vi "FPGAcode2_test.vi"() -> ()   [LabVIEW 2015]
uses:
  <vilib>/Platform/TimedLoop/XDataNode/timing_clust.ctl
  <vilib>/Platform/TimedLoop/XDataNode/nitl_modes.ctl
  <vilib>/Platform/TimedLoop/XDataNode/wakeup.ctl
  <vilib>/rvi/Emulation/niFpgaGetClockAttributes.vi
  <vilib>/rvi/Emulation/niFpgaSctlEmulationGetInTimedLoop.vi
  <vilib>/rvi/Emulation/niFpgaEmulationReportErrorSimple.vi
  <vilib>/rvi/Emulation/niFpgaProcessEmulError.vi
  <vilib>/rvi/eio/common/nirviEmuTemplateMethod_errors.vi
  <vilib>/rvi/Emulation/niFpgaCriticalErrorInLSC.vi
  <vilib>/eio/EIONode/EIONode.xnode
  <vilib>/Platform/TimedLoop/XDataNode/XDataNode.xnode
  <vilib>/Platform/TimedLoop/XDataNode/XDNodeRunTimeDep.lvlib
panel:
  out "New Average":T1
  in  "Cluster":T1
  out "Detector 3 Correlation 7":i16
  out "Detector 3 Correlation 6":i16
  out "Detector 3 Correlation 5":i16
  out "Detector 3 Correlation 4":i16
  out "Detector 3 Correlation 3":i16
  out "Detector 3 Correlation 2":i16
  out "Detector 3 Correlation 1":i16
  out "Detector 1 Correlation 7":i16
  out "Detector 1 Correlation 6":i16
  out "Detector 1 Correlation 5":i16
  out "Detector 1 Correlation 4":i16
  out "Detector 1 Correlation 3":i16
  out "Detector 1 Correlation 2":i16
  out "Detector 1 Correlation 1":i16
  in  "Filter threshold 7":i32=1000
  in  "Filter threshold 6":i32=1000
  in  "Filter threshold 5":i32=1000
  in  "Filter threshold 4":i32=1000
  in  "Filter threshold 3":i32=1000
  in  "Filter threshold 2":i32=1000
  in  "Filter threshold 1":i32=1000
  out "Del Armed":bool
  out "Armed":bool
  out "Delay":bool
  out "Plates":bool
  in  "Reset One Shot":bool
  in  "One Shot":bool
  in  "High Charge Limit":i16
  in  "Low Charge Limit":i16
  in  "High Velocity Count":i32
  in  "Low Velocity Count":i32
  in  "High Mass Limit":i64
  in  "Low Mass Limit":i64
  in  "Mult1":fxp<+,16,7>
  out "IO Module\\AI 0":i16
  out "IO Module\\AI 1":i16
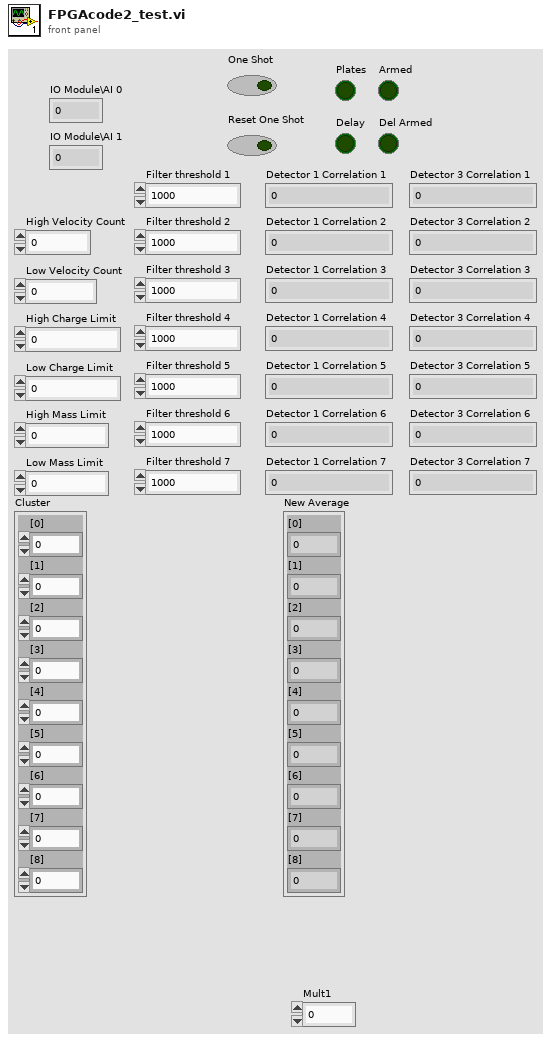
[diagram p1: front panel]
types:
  T1 = cluster{"[0]":i32, "[1]":i32, "[2]":i32, "[3]":i32, "[4]":i32, "[5]":i32, "[6]":i32, "[7]":i32, "[8]":i32}
  T2 = typedef "XDNodeRunTimeDep.lvlib/timing_clust.ctl" = cluster{"Expected End [f-1]":u64, "Actual End [f-1]":u64, "Finished Late? [f-1]":bool, "Expected End [i-1]":u64, "Actual End [i-1]":u64, "Finished Late? [i-1]":bool, "Expected Start [i]":u64, "Actual Start [i]":u64, "Expected Start [f]":u64, "Actual Start [f]":u64, "Source Name":string, "Structure Name":string, "Period":i64, "Deadline":i64, "Offset":i64, "Start":i64, "Priority":i32, "Timeout":i32, "Mode":T3, "Wakeup Reason":T4, "Error":errorcluster, "Source Type":string, "Secondary Source Type":string, "Global End Time":u64, "Global Start Time":u64, "Frame Duration":u64, "Iteration Duration":u64, "Assigned CPU":i32, "I/O Scan Engine Mode":u32}
  T3 = typedef "XDNodeRunTimeDep.lvlib/nitl_modes.ctl" = enum32{"No Change", "Process missed periods, maintain original phase", "Discard missed periods, maintain original phase", "Process missed periods, ignore original phase", "Discard missed periods, ignore original phase"}
  T4 = typedef "XDNodeRunTimeDep.lvlib/wakeup.ctl" = enum32{"Normal", "Aborted", "Asynchronous wakeup", "Timing source error", "Timed loop error", "Timeout"}
  T5 = cluster{"[0]":u8, "[1]":u8, "[2]":u8, "[3]":u8, "[4]":u8, "[5]":u8, "[6]":u8, "[7]":u8, "[8]":u8}
  T6 = cluster{"High Charge Limit":i16, "Low Charge Limit":i16, "Time Out Limit":i32, "High Velocity Count":i32, "Low Velocity Count":i32, "Sampling Rate":fxp<+,30,25>, "High Mass Limit":i64, "Low Mass Limit":i64}
  T7 = cluster{"[0]":u32, "[1]":u32, "[2]":u32, "[3]":u32, "[4]":u32, "[5]":u32, "[6]":u32, "[7]":u32, "[8]":u32}
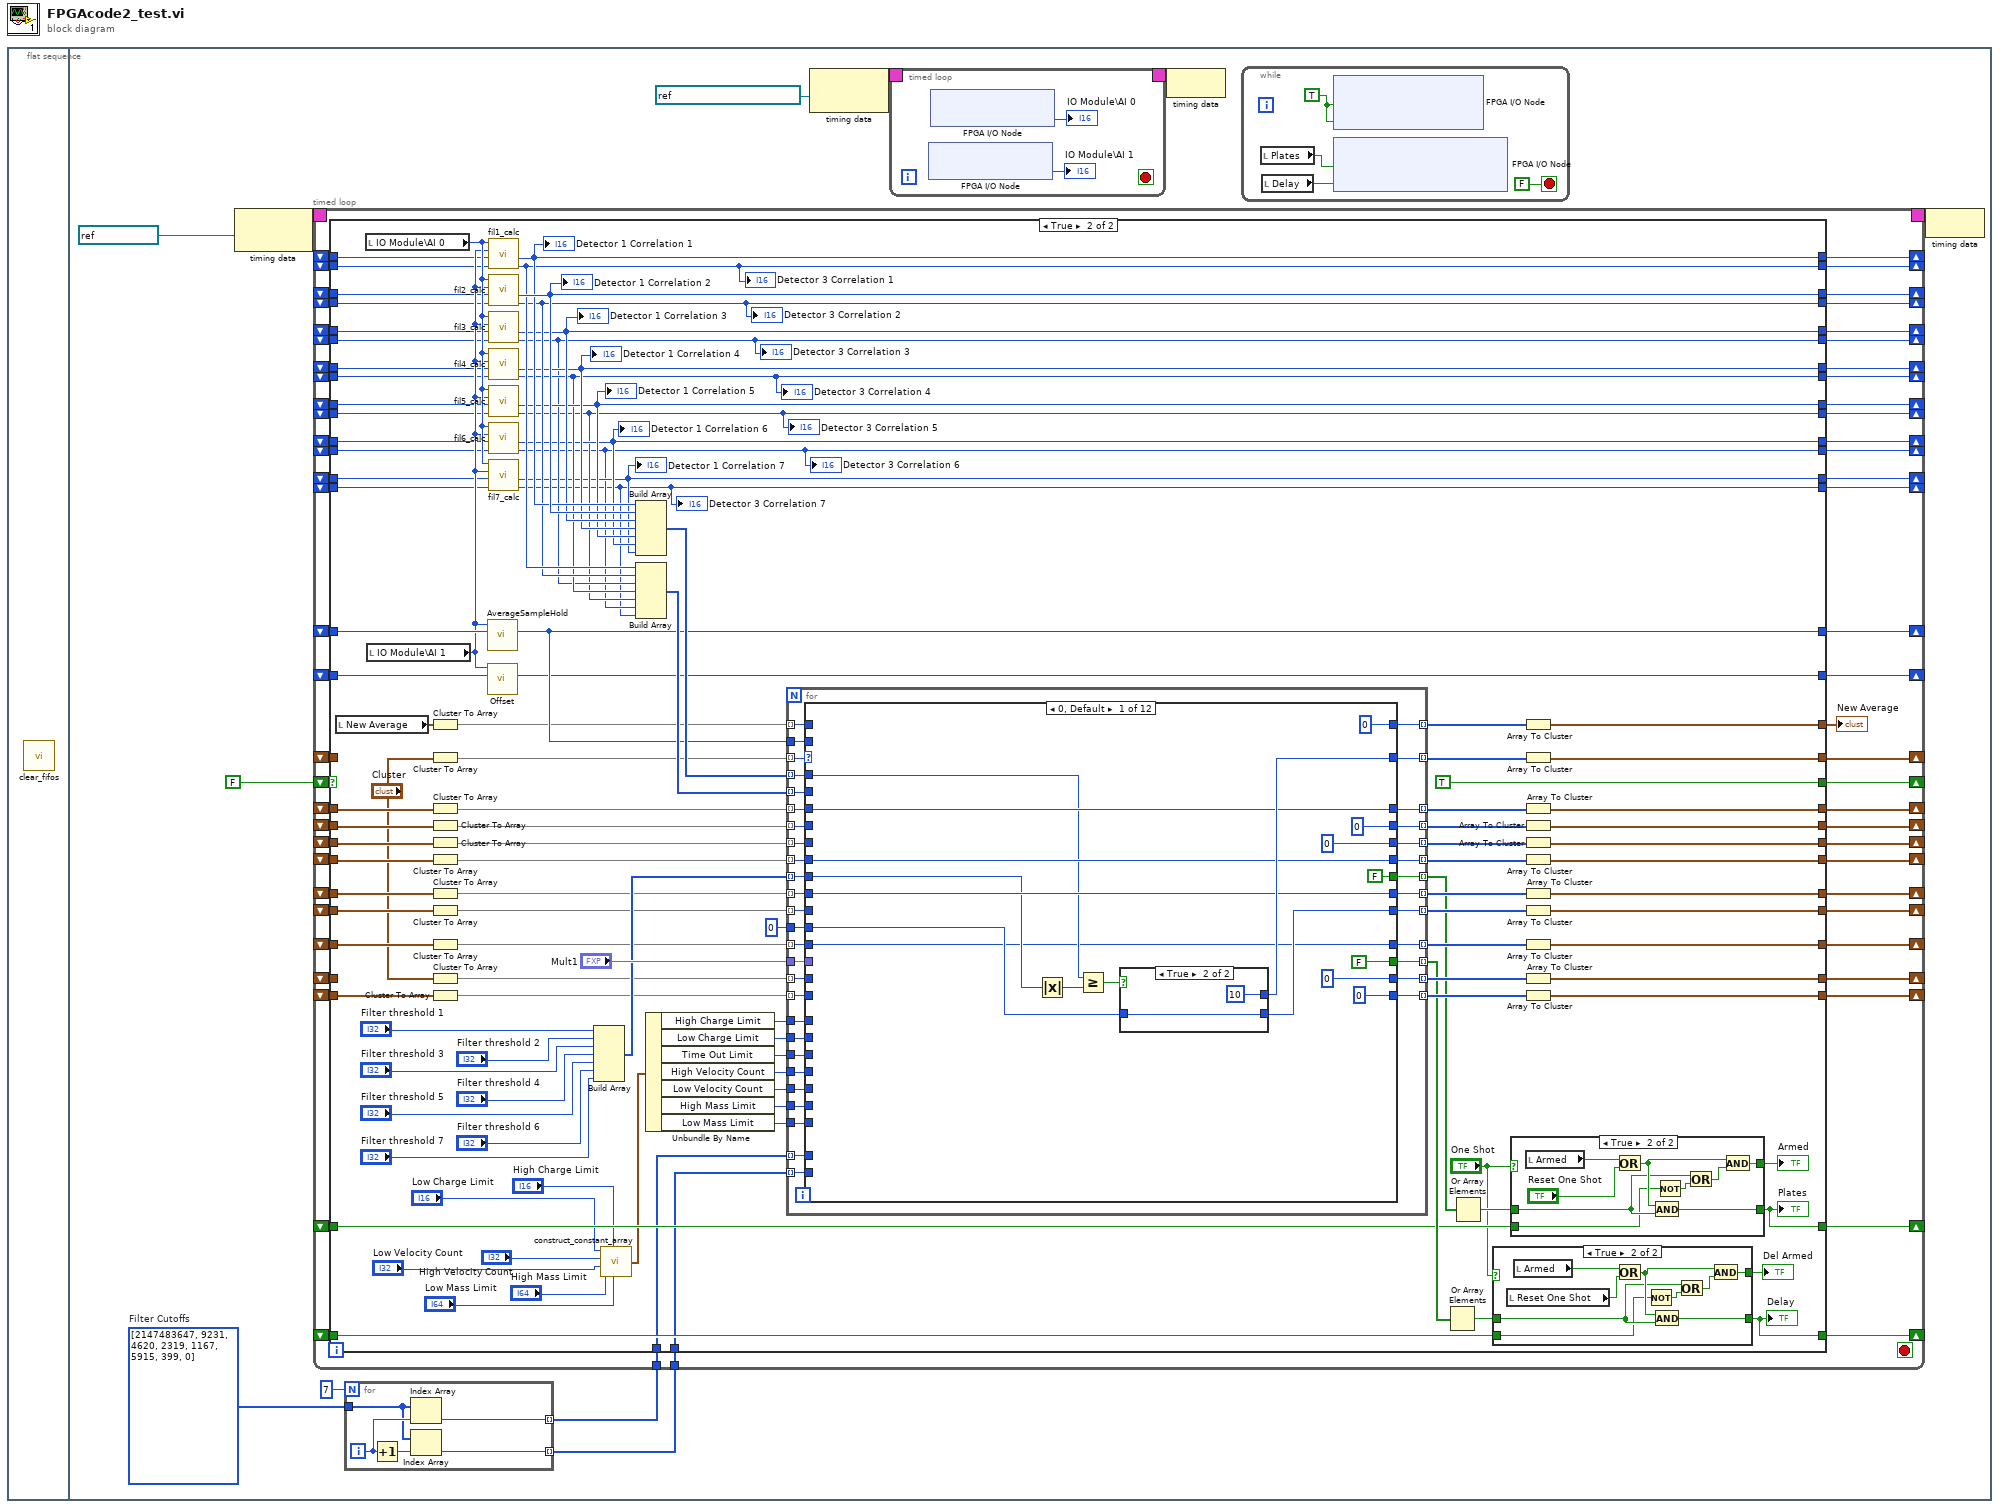
[diagram p0: block diagram]
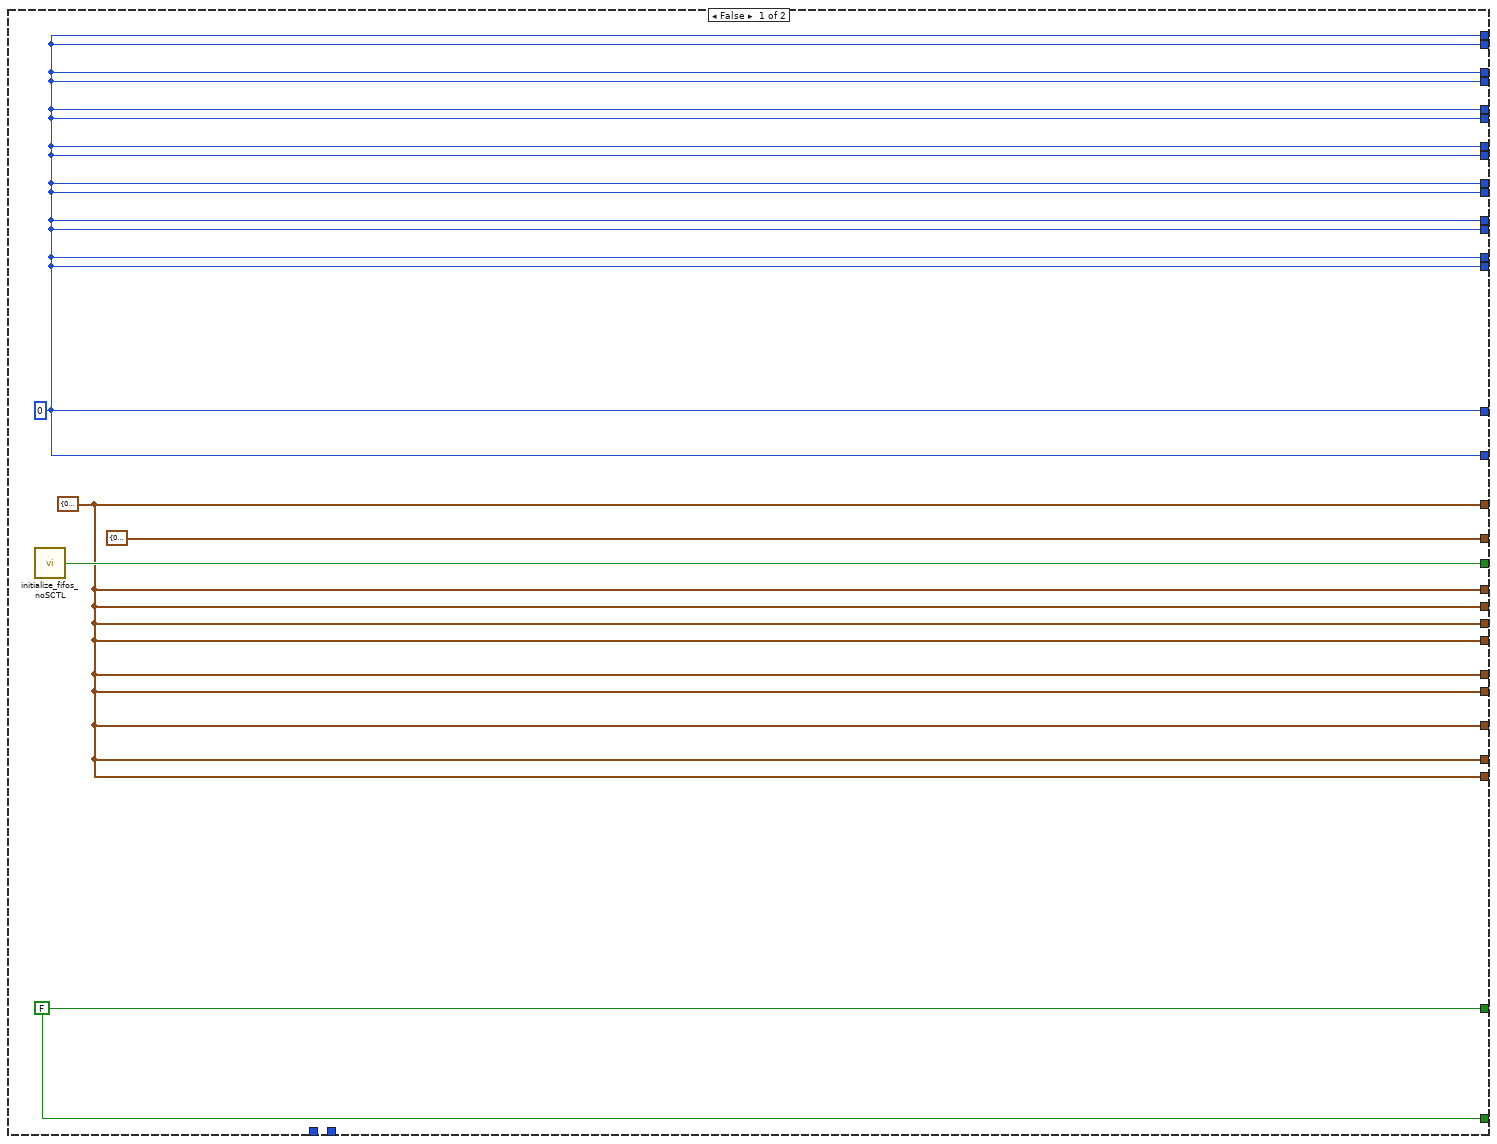
[diagram p2: hidden frame]
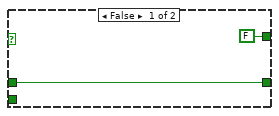
[diagram p3: hidden frame]
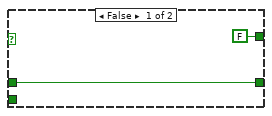
[diagram p4: hidden frame]
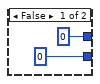
[diagram p5: hidden frame]
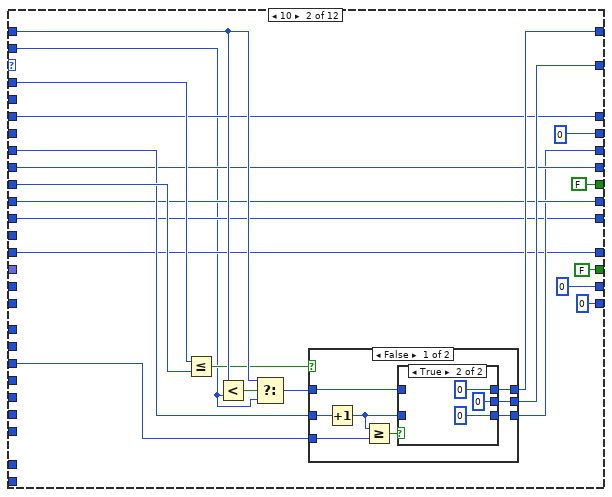
[diagram p6: hidden frame]
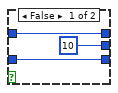
[diagram p7: hidden frame]
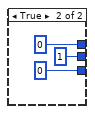
[diagram p8: hidden frame]
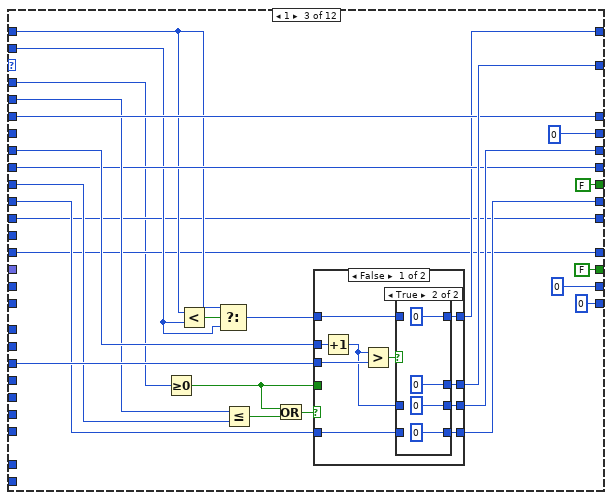
[diagram p9: hidden frame]
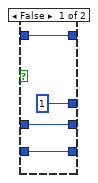
[diagram p10: hidden frame]
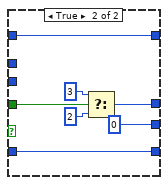
[diagram p11: hidden frame]
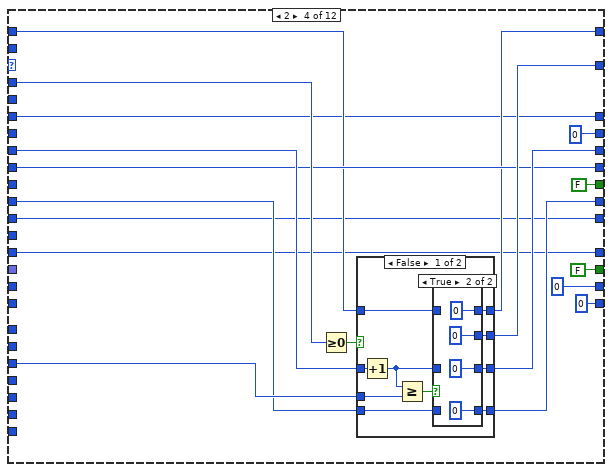
[diagram p12: hidden frame]
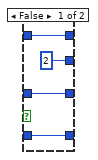
[diagram p13: hidden frame]
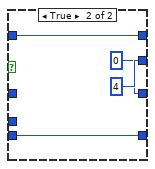
[diagram p14: hidden frame]
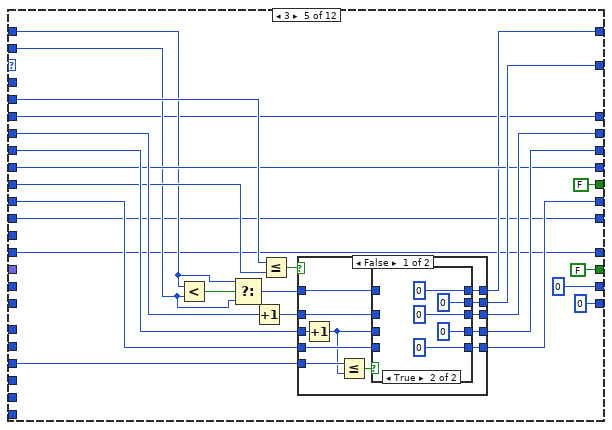
[diagram p15: hidden frame]
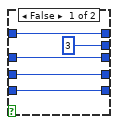
[diagram p16: hidden frame]
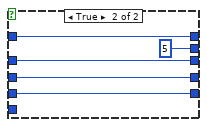
[diagram p17: hidden frame]
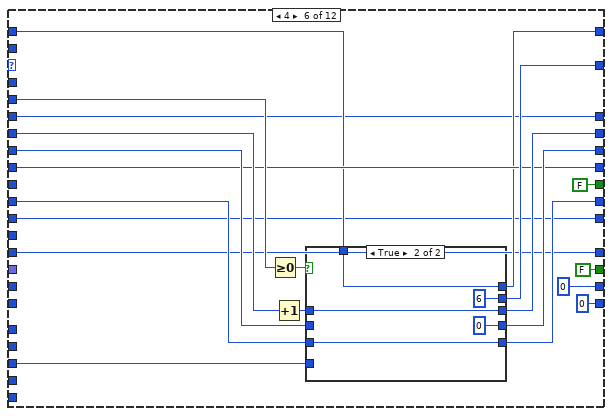
[diagram p18: hidden frame]
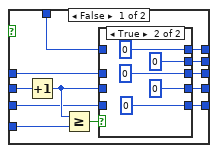
[diagram p19: hidden frame]
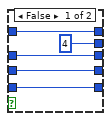
[diagram p20: hidden frame]
diagram:
  n1 = flat-sequence {
    frame #0 {
      n2 = call "clear_fifos.vi"() -> ()  [unwired: 1 in]
    }
    frame #1 {
      w3 = i32[] [2147483647, 9231, 4620, 2319, 1167, 5915, 399, 0]  # Filter Cutoffs
      n3 = node-c288(refnum<k21> "26.67MHz" ("Source Name")) -> (w11:T2)
      n4 = for {
        N: 7 -> [_]
        tunnel: w3 -> [w14]
        tunnel: [w13] -> w2 mode=indexing
        tunnel: [w12] -> w1 mode=indexing
        i -> [w16]
        n5 = Increment(x=w16) -> (x+1=w15:i32)
        n6 = Index Array(array=w14, index=w16) -> (element=w13:i32)
        n7 = Index Array(array=w14, index=w15) -> (element=w12:i32)
      }
      n8 = timed-loop {
        timing: w11 -> [_]
        timing-out: [_] -> w10
        shift-right: [w88] -> _
        shift-left: FALSE -> [w89]
        shift-right: [w86] -> _
        shift-left: _ -> [w87]
        shift-right: [w84] -> _
        shift-left: _ -> [w85]
        shift-right: [w70] -> _
        shift-left: _ -> [w83]
        shift-right: [w81] -> _
        shift-left: _ -> [w82]
        shift-right: [w79] -> _
        shift-left: _ -> [w80]
        shift-right: [w69] -> _
        shift-left: _ -> [w78]
        shift-right: [w68] -> _
        shift-left: _ -> [w77]
        shift-right: [w64] -> _
        shift-left: _ -> [w76]
        shift-right: [w74] -> _
        shift-left: _ -> [w75]
        shift-right: [w67] -> _
        shift-left: _ -> [w73]
        shift-right: [w66] -> _
        shift-left: _ -> [w72]
        shift-right: [w65] -> _
        shift-left: _ -> [w71]
        shift-right: [w63] -> _
        shift-left: _ -> [w62]
        shift-right: [w60] -> _
        shift-left: _ -> [w61]
        shift-right: [w59] -> _
        shift-left: _ -> [w58]
        shift-right: [w57] -> _
        shift-left: _ -> [w56]
        shift-right: [w55] -> _
        shift-left: _ -> [w51]
        shift-right: [w54] -> _
        shift-left: _ -> [w50]
        shift-right: [w53] -> _
        shift-left: _ -> [w49]
        shift-right: [w52] -> _
        shift-left: _ -> [w48]
        shift-right: [w47] -> _
        shift-left: _ -> [w39]
        shift-right: [w46] -> _
        shift-left: _ -> [w38]
        shift-right: [w45] -> _
        shift-left: _ -> [w37]
        shift-right: [w44] -> _
        shift-left: _ -> [w32]
        shift-right: [w43] -> _
        shift-left: _ -> [w36]
        shift-right: [w42] -> _
        shift-left: _ -> [w33]
        shift-right: [w41] -> _
        shift-left: _ -> [w35]
        shift-right: [w40] -> _
        shift-left: _ -> [w34]
        tunnel: w2 -> [w31]
        tunnel: w1 -> [w30]
        stop <- _ stop-if-true
        n9 = case shown="True" w89 {
          tunnel: [w94 TRUE] -> w88
          tunnel: [w90 w121] -> w29
          tunnel: w87 -> [_ w209]
          tunnel: [w92 w146] -> w86
          tunnel: w85 -> [_ _]
          tunnel: [T5 {"[0]"=0, "[1]"=0, "[2]"=0, "[3]"=0, "[4]"=0, "[5]"=0, "[6]"=0, "[7]"=0, "[8]"=0} w120] -> w84
          tunnel: w83 -> [_ w207]
          tunnel: w82 -> [_ w97]
          tunnel: [w90 w111] -> w81
          tunnel: w80 -> [_ _]
          tunnel: [w90 w112] -> w79
          tunnel: w78 -> [_ w204]
          tunnel: w77 -> [_ w203]
          tunnel: w76 -> [_ w202]
          tunnel: w75 -> [_ w201]
          tunnel: [w92 w99] -> w74
          tunnel: w73 -> [_ w200]
          tunnel: w72 -> [_ w199]
          tunnel: w71 -> [_ w198]
          tunnel: [w90 w119] -> w70
          tunnel: [w90 w118] -> w69
          tunnel: [w90 w117] -> w68
          tunnel: [w90 w116] -> w67
          tunnel: [w90 w115] -> w66
          tunnel: [w90 w114] -> w65
          tunnel: [w90 w113] -> w64
          tunnel: [w93 w185] -> w63
          tunnel: w62 -> [_ w186]
          tunnel: w61 -> [_ w182]
          tunnel: [w93 w181] -> w60
          tunnel: [w92 w132] -> w59
          tunnel: w58 -> [_ w160]
          tunnel: [w92 w134] -> w57
          tunnel: w56 -> [_ w159]
          tunnel: [w92 w133] -> w55
          tunnel: [w92 w136] -> w54
          tunnel: [w92 w135] -> w53
          tunnel: [w92 w139] -> w52
          tunnel: w51 -> [_ w158]
          tunnel: w50 -> [_ w157]
          tunnel: w49 -> [_ w156]
          tunnel: w48 -> [_ w155]
          tunnel: [w92 w138] -> w47
          tunnel: [w92 w140] -> w46
          tunnel: [w92 w137] -> w45
          tunnel: [w92 w141] -> w44
          tunnel: [w92 w142] -> w43
          tunnel: [w92 w145] -> w42
          tunnel: [w92 w143] -> w41
          tunnel: [w92 w144] -> w40
          tunnel: w39 -> [_ w154]
          tunnel: w38 -> [_ w153]
          tunnel: w37 -> [_ w152]
          tunnel: w36 -> [_ w151]
          tunnel: w35 -> [_ w150]
          tunnel: w34 -> [_ w149]
          tunnel: w33 -> [_ w148]
          tunnel: w32 -> [_ w147]
          tunnel: w31 -> [_ w131]
          tunnel: w30 -> [_ w130]
          frame False {
            w90 = T1 {"[0]"=0, "[1]"=0, "[2]"=0, "[3]"=0, "[4]"=0, "[5]"=0, "[6]"=0, "[7]"=0, "[8]"=0}
            w93 = FALSE
            w92 = i16 0 ("Output New Average")
            n10 = call "initialize_fifos_noSCTL.vi"() -> ("Output State"=w94:bool)
          }
          frame True {
            n11 = local read "New Average"() -> (w95:T1)
            n12 = local read "IO Module\\AI 0"() -> (w172:i16)
            n13 = local read "IO Module\\AI 1"() -> (w171:i16)
            n14 = Cluster To Array(cluster=w95) -> (array=w110:i32[])
            n15 = Cluster To Array(cluster="Cluster") -> (array=w109:i32[])
            n16 = Cluster To Array(cluster=w207) -> (array=w108:i32[])
            n17 = Cluster To Array(cluster=w204) -> (array=w107:i32[])
            n18 = Cluster To Array(cluster=w203) -> (array=w106:u32[])
            n19 = Cluster To Array(cluster=w200) -> (array=w105:i32[])
            n20 = Cluster To Array(cluster=w199) -> (array=w104:i32[])
            n21 = Cluster To Array(cluster=w198) -> (array=w103:i32[])
            n22 = Cluster To Array(cluster=w202) -> (array=w102:i32[])
            n23 = Cluster To Array(cluster="Cluster") -> (array=w101:i32[])
            n24 = Cluster To Array(cluster=w97) -> (array=w100:i32[])
            n25 = call "AverageSampleHold.vi"("Previous Average"=w209, "Input Value"=w171) -> ("Output New Average"=w146:i16)  [unwired: 9 in]
            n26 = call "Offset.vi"("Previous Average"=w201, "Input Value"=w171) -> ("Output New Average"=w99:i16)  [unwired: 9 in]
            n27 = call "fil1_calc.vi"("Detector 3 Correlation In"=w150, "Detector 1 Correlation In"=w149, "AI1"=w171, "AI0"=w172) -> ("Detector 3 Correlation Out"=w143:i16, "Detector 1 Correlation Out"=w144:i16)  [unwired: 4 in]
            "Detector 1 Correlation 1" <- w144
            "Detector 3 Correlation 1" <- w143
            n28 = call "fil2_calc.vi"("Detector 3 Correlation In"=w151, "Detector 1 Correlation In"=w148, "AI1"=w171, "AI0"=w172) -> ("Detector 3 Correlation Out"=w142:i16, "Detector 1 Correlation Out"=w145:i16)  [unwired: 4 in]
            "Detector 1 Correlation 2" <- w145
            "Detector 3 Correlation 2" <- w142
            n29 = call "fil3_calc.vi"("Detector 3 Correlation In"=w152, "Detector 1 Correlation In"=w147, "AI1"=w171, "AI0"=w172) -> ("Detector 3 Correlation Out"=w137:i16, "Detector 1 Correlation Out"=w141:i16)  [unwired: 4 in]
            "Detector 1 Correlation 3" <- w141
            "Detector 3 Correlation 3" <- w137
            n30 = call "fil4_calc.vi"("Detector 3 Correlation In"=w154, "Detector 1 Correlation In"=w153, "AI1"=w171, "AI0"=w172) -> ("Detector 3 Correlation Out"=w138:i16, "Detector 1 Correlation Out"=w140:i16)  [unwired: 4 in]
            "Detector 1 Correlation 4" <- w140
            "Detector 3 Correlation 4" <- w138
            n31 = call "fil5_calc.vi"("Detector 3 Correlation In"=w156, "Detector 1 Correlation In"=w155, "AI1"=w171, "AI0"=w172) -> ("Detector 3 Correlation Out"=w135:i16, "Detector 1 Correlation Out"=w139:i16)  [unwired: 4 in]
            "Detector 1 Correlation 5" <- w139
            "Detector 3 Correlation 5" <- w135
            n32 = call "fil6_calc.vi"("Detector 3 Correlation In"=w158, "Detector 1 Correlation In"=w157, "AI1"=w171, "AI0"=w172) -> ("Detector 3 Correlation Out"=w133:i16, "Detector 1 Correlation Out"=w136:i16)  [unwired: 4 in]
            "Detector 1 Correlation 6" <- w136
            "Detector 3 Correlation 6" <- w133
            n33 = call "fil7_calc.vi"("Detector 3 Correlation In"=w160, "Detector 1 Correlation In"=w159, "AI1"=w171, "AI0"=w172) -> ("Detector 3 Correlation Out"=w132:i16, "Detector 1 Correlation Out"=w134:i16)  [unwired: 4 in]
            "Detector 1 Correlation 7" <- w134
            "Detector 3 Correlation 7" <- w132
            n34 = Build Array("Filter threshold 1", "Filter threshold 2", "Filter threshold 3", "Filter threshold 4", "Filter threshold 5", "Filter threshold 6", "Filter threshold 7") -> (w161:i32[])
            n35 = call "construct_constant_array.vi"("Low Mass Limit"="Low Mass Limit", "High Charge Limit"="High Charge Limit", "High Mass Limit"="High Mass Limit", "Low Velocity Count"="Low Velocity Count", "High Velocity Count"="High Velocity Count", "Low Charge Limit"="Low Charge Limit") -> ("Limits"=w129:T6)
            n36 = Build Array(w144, w145, w141, w140, w139, w136, w134) -> (w170:i16[])
            n37 = Build Array(w143, w142, w137, w138, w135, w133, w132) -> (w169:i16[])
            n38 = Unbundle By Name(w129) -> ("High Charge Limit"=w122:i16, "Low Charge Limit"=w123:i16, "Time Out Limit"=w124:i32, "High Velocity Count"=w125:i32, "Low Velocity Count"=w126:i32, "High Mass Limit"=w127:i64, "Low Mass Limit"=w128:i64)
            n39 = for {
              tunnel: w170 -> [w269] mode=indexing
              tunnel: w169 -> [w268] mode=indexing
              tunnel: w110 -> [w272] mode=indexing
              tunnel: [w253] -> w210 mode=indexing
              tunnel: w109 -> [w270] mode=indexing
              tunnel: [w252] -> w208 mode=indexing
              tunnel: w108 -> [w267] mode=indexing
              tunnel: w100 -> [w256] mode=indexing
              tunnel: [w241] -> w206 mode=indexing
              tunnel: w101 -> [w257] mode=indexing
              tunnel: [w242] -> w205 mode=indexing
              tunnel: w107 -> [w266] mode=indexing
              tunnel: w106 -> [w265] mode=indexing
              tunnel: w102 -> [w259] mode=indexing
              tunnel: w105 -> [w264] mode=indexing
              tunnel: w161 -> [w263] mode=indexing
              tunnel: w104 -> [w262] mode=indexing
              tunnel: w103 -> [w261] mode=indexing
              tunnel: [w251] -> w197 mode=indexing
              tunnel: [w250] -> w196 mode=indexing
              tunnel: [w249] -> w195 mode=indexing
              tunnel: [w248] -> w194 mode=indexing
              tunnel: [w245] -> w193 mode=indexing
              tunnel: [w244] -> w192 mode=indexing
              tunnel: [w243] -> w191 mode=indexing
              tunnel: [w247] -> w190 mode=indexing
              tunnel: [w246] -> w189 mode=indexing
              tunnel: "Mult1" -> [w258]
              tunnel: w146 -> [w271]
              tunnel: i16 0 ("Output New Average") -> [w260]
              tunnel: w131 -> [w255] mode=indexing
              tunnel: w130 -> [w254] mode=indexing
              tunnel: w128 -> [w240]
              tunnel: w127 -> [w239]
              tunnel: w126 -> [w238]
              tunnel: w125 -> [w237]
              tunnel: w124 -> [w236]
              tunnel: w123 -> [w235]
              tunnel: w122 -> [w234]
              n40 = case shown="0, Default" w270 {
                tunnel: w269 -> [w283 w314 w334 w399 _ _ _ _ _ _ _ _]
                tunnel: w268 -> [_ _ w351 _ w442 w490 w537 _ _ _ _ _]
                tunnel: w263 -> [w281 w313 w350 _ w441 _ _ _ _ _ _ _]
                tunnel: w266 -> [_ _ _ _ w444 w498 w546 w589 w646 w675 w705 _]
                tunnel: [0 0 0 0 w450 w496 w539 w574 w645 w673 w703 0] -> w250
                tunnel: [w290 w311 w359 w403 w449 w493 w542 w594 w644 w674 w704 w729] -> w252
                tunnel: w267 -> [w287 w306 w352 w390 w430 w482 w538 w595 w620 w659 w701 w720]
                tunnel: w236 -> [_ w309 w358 w402 w447 w491 w543 _ _ _ _ _]
                tunnel: w265 -> [_ w310 w357 w401 w448 w492 w545 _ _ _ _ _]
                tunnel: [u32 0 w301 w356 w400 w446 w494 w541 u32 0 u32 0 ("Timeout Count in") u32 0 ("Timeout Count in") u32 0 u32 0 ("Timeout Count in")] -> w249
                tunnel: w238 -> [_ _ _ _ _ _ _ _ w643 _ _ _]
                tunnel: w237 -> [_ _ _ _ _ _ _ _ w642 _ _ _]
                tunnel: [w287 w306 w352 w390 w430 w482 w538 w596 w620 w659 w701 w720] -> w251
                tunnel: w235 -> [_ _ _ _ _ _ _ _ w641 _ _ _]
                tunnel: w234 -> [_ _ _ _ _ _ _ _ w640 _ _ _]
                tunnel: w262 -> [w286 w303 w349 w397 w440 w485 w536 w592 w639 w671 w699 _]
                tunnel: [w286 w303 w348 w396 w439 w489 w535 w593 w638 w671 w700 0 ("Noise Level")] -> w245
                tunnel: w264 -> [w285 w304 w347 w395 w438 w488 w534 w591 w621 w667 w696 w722]
                tunnel: [w285 w304 w347 w395 w438 w488 w534 w591 w621 w668 w696 w722] -> w248
                tunnel: [0 ("Old Average In") w307 w346 w394 w437 w487 w533 w590 w634 w664 0 ("Old Average In") 0 ("Old Average In")] -> w253
                tunnel: w255 -> [_ _ _ _ _ _ _ w576 _ _ _ _]
                tunnel: w254 -> [_ _ _ _ _ _ _ w575 _ _ _ _]
                tunnel: [FALSE FALSE ("Data") FALSE FALSE FALSE FALSE FALSE FALSE FALSE ("Data") w658 w690 FALSE ("Data")] -> w247
                tunnel: w272 -> [_ w315 w343 w392 w434 w484 w531 w586 w634 w664 _ _]
                tunnel: w271 -> [_ w295 w342 _ w433 _ _ _ _ _ _ _]
                tunnel: w261 -> [_ w300 w340 w391 w431 w483 w530 w585 w635 w663 _ _]
                tunnel: w260 -> [w278 _ _ _ _ _ _ _ _ _ _ _]
                tunnel: [w279 w300 w340 w391 w431 w483 w530 w585 w635 w663 0 ("Offset") 0 ("Offset")] -> w244
                tunnel: [w277 w299 w339 w389 w429 w481 w529 w584 w622 w669 w694 w727] -> w243
                tunnel: w259 -> [w277 w299 w339 w389 w429 w481 w529 w584 w622 w670 w694 w727]
                tunnel: w239 -> [_ _ _ _ _ _ _ _ w633 _ _ _]
                tunnel: w240 -> [_ _ _ _ _ _ _ _ w632 _ _ _]
                tunnel: w257 -> [_ _ _ _ _ _ _ _ w628 w662 w693 w718]
                tunnel: [0 0 0 0 0 0 0 w580 w627 w660 w688 w715] -> w241
                tunnel: [FALSE FALSE FALSE FALSE FALSE FALSE FALSE FALSE FALSE w657 w689 w719] -> w246
                tunnel: [u16 0 u16 0 u16 0 u16 0 u16 0 u16 0 u16 0 u16 0 u16 0 u16 0 w692 w728] -> w242
                tunnel: w256 -> [_ _ _ _ _ _ _ _ _ _ _ w716]
                tunnel: w258 -> [_ _ _ _ _ _ _ w579 _ _ _ _]
                frame 0, Default {
                  n41 = Absolute Value(x=w281) -> (abs(x)=w280:i32)
                  n42 = Greater Or Equal?(x=w283, y=w280) -> (x >= y?=w288:bool)
                  n43 = case shown="True" w288 {
                    tunnel: [u8 0 u8 10] -> w290
                    tunnel: [0 w293] -> w279
                    tunnel: w278 -> [_ w293]
                    frame False {
                    }
                    frame True {
                    }
                  }
                }
                frame 10 {
                  n44 = Less Or Equal?(x=w314, y=w313) -> (x <= y?=w312:bool)
                  n45 = Less?(x=w315, y=w295) -> (x < y?=w316:bool)
                  n46 = Select(t=w315, s=w316, f=w295) -> (s? t:f=w308:i32)
                  n47 = case shown="False" w312 {
                    tunnel: [w322 u8 1] -> w311
                    tunnel: w310 -> [w319 _]
                    tunnel: w309 -> [w324 _]
                    tunnel: w308 -> [w321 _]
                    tunnel: [w320 0 ("New Average")] -> w307
                    tunnel: [w317 0] -> w301
                    frame False {
                      n48 = Increment(x=w319) -> (x+1=w318:u32)
                      n49 = Greater Or Equal?(x=w318, y=w324) -> (x >= y?=w323:bool)
                      n50 = case shown="True" w323 {
                        tunnel: [u8 10 u8 0] -> w322
                        tunnel: w321 -> [w327 _]
                        tunnel: [w327 0 ("New Average")] -> w320
                        tunnel: w318 -> [w325 _]
                        tunnel: [w325 0] -> w317
                        frame False {
                        }
                        frame True {
                        }
                      }
                    }
                    frame True {
                    }
                  }
                }
                frame 1 {
                  n51 = Greater Or Equal To 0?(x=w334) -> (x >= 0?=w354:bool)
                  n52 = Less?(x=w343, y=w342) -> (x < y?=w344:bool)
                  n53 = Select(t=w343, s=w344, f=w342) -> (s? t:f=w341:i32)
                  n54 = Less Or Equal?(x=w351, y=w350) -> (x <= y?=w353:bool)
                  n55 = Or(x=w354, y=w353) -> (x .or. y?=w355:bool)
                  n56 = case shown="False" w355 {
                    tunnel: [w367 w378] -> w359
                    tunnel: w358 -> [w369 _]
                    tunnel: w357 -> [w366 _]
                    tunnel: [w365 u32 0] -> w356
                    tunnel: w354 -> [_ w379]
                    tunnel: w349 -> [w364 w383]
                    tunnel: [w363 w383] -> w348
                    tunnel: [w362 w384] -> w346
                    tunnel: w341 -> [w360 w384]
                    frame False {
                      n57 = Increment(x=w366) -> (x+1=w361:u32)
                      n58 = Greater?(x=w361, y=w369) -> (0:w368:bool)
                      n59 = case shown="True" w368 {
                        tunnel: [u8 1 u8 0 ("Old Average In")] -> w367
                        tunnel: w361 -> [w372 _]
                        tunnel: [w372 u32 0 ("Old Average In")] -> w365
                        tunnel: w364 -> [w371 _]
                        tunnel: [w371 0 ("Old Average In")] -> w363
                        tunnel: [w370 0 ("Old Average In")] -> w362
                        tunnel: w360 -> [w370 _]
                        frame False {
                        }
                        frame True {
                        }
                      }
                    }
                    frame True {
                      n60 = Select(t=u8 3, s=w379, f=u8 2) -> (s? t:f=w378:u8)
                    }
                  }
                }
                frame 2 {
                  n61 = Greater Or Equal To 0?(x=w399) -> (x >= 0?=w398:bool)
                  n62 = case shown="False" w398 {
                    tunnel: [w412 u8 4] -> w403
                    tunnel: w402 -> [w411 _]
                    tunnel: w401 -> [w409 _]
                    tunnel: [w410 u32 0] -> w400
                    tunnel: w397 -> [w408 w423]
                    tunnel: [w407 w423] -> w396
                    tunnel: [w406 w422] -> w394
                    tunnel: w392 -> [w405 w422]
                    frame False {
                      n63 = Increment(x=w409) -> (x+1=w404:u32)
                      n64 = Greater Or Equal?(x=w404, y=w411) -> (x >= y?=w413:bool)
                      n65 = case shown="True" w413 {
                        tunnel: [u8 2 u8 0] -> w412
                        tunnel: w404 -> [w417 _]
                        tunnel: [w417 u32 0] -> w410
                        tunnel: w408 -> [w415 _]
                        tunnel: [w415 0 ("High Correlation In")] -> w407
                        tunnel: [w414 0 ("Old Average In")] -> w406
                        tunnel: w405 -> [w414 _]
                        frame False {
                        }
                        frame True {
                        }
                      }
                    }
                    frame True {
                    }
                  }
                }
                frame 3 {
                  n66 = Less?(x=w434, y=w433) -> (x < y?=w435:bool)
                  n67 = Select(t=w434, s=w435, f=w433) -> (s? t:f=w432:i32)
                  n68 = Increment(x=w444) -> (x+1=w443:i32)
                  n69 = Less Or Equal?(x=w442, y=w441) -> (x <= y?=w445:bool)
                  n70 = case shown="False" w445 {
                    tunnel: w443 -> [w458 w477]
                    tunnel: [w457 w477] -> w450
                    tunnel: [w460 u8 5] -> w449
                    tunnel: w448 -> [w456 w473]
                    tunnel: w447 -> [w462 _]
                    tunnel: [w459 w473] -> w446
                    tunnel: w440 -> [w455 w475]
                    tunnel: [w454 w475] -> w439
                    tunnel: [w453 w474] -> w437
                    tunnel: w432 -> [w452 w474]
                    frame False {
                      n71 = Increment(x=w456) -> (x+1=w451:u32)
                      n72 = Less Or Equal?(x=w462, y=w451) -> (x <= y?=w461:bool)
                      n73 = case shown="True" w461 {
                        tunnel: [u8 3 u8 0] -> w460
                        tunnel: w451 -> [w466 _]
                        tunnel: [w466 u32 0] -> w459
                        tunnel: w458 -> [w465 _]
                        tunnel: [w465 0] -> w457
                        tunnel: w455 -> [w464 _]
                        tunnel: [w464 0 ("High Correlation In")] -> w454
                        tunnel: [w463 0 ("Old Average In")] -> w453
                        tunnel: w452 -> [w463 _]
                        frame False {
                        }
                        frame True {
                        }
                      }
                    }
                    frame True {
                    }
                  }
                }
                frame 4 {
                  n74 = Greater Or Equal To 0?(x=w490) -> (x >= 0?=w497:bool)
                  n75 = Increment(x=w498) -> (x+1=w495:i32)
                  n76 = case shown="True" w497 {
                    tunnel: [w503 w525] -> w496
                    tunnel: w495 -> [w504 w525]
                    tunnel: [w506 u32 0] -> w494
                    tunnel: [w508 u8 6] -> w493
                    tunnel: w492 -> [w510 _]
                    tunnel: w491 -> [w505 _]
                    tunnel: w485 -> [w502 w522]
                    tunnel: [w501 w522] -> w489
                    tunnel: [w500 w521] -> w487
                    tunnel: w484 -> [w499 w521]
                    frame False {
                      n77 = Increment(x=w510) -> (x+1=w507:u32)
                      n78 = Greater Or Equal?(x=w507, y=w505) -> (x >= y?=w509:bool)
                      n79 = case shown="True" w509 {
                        tunnel: [u8 4 u8 0] -> w508
                        tunnel: w507 -> [w514 _]
                        tunnel: [w514 u32 0] -> w506
                        tunnel: w504 -> [w513 _]
                        tunnel: [w513 0] -> w503
                        tunnel: w502 -> [w512 _]
                        tunnel: [w512 0 ("High Correlation In")] -> w501
                        tunnel: [w511 0 ("Old Average In")] -> w500
                        tunnel: w499 -> [w511 _]
                        frame False {
                        }
                        frame True {
                        }
                      }
                    }
                    frame True {
                    }
                  }
                }
                frame 5 {
                  n80 = Increment(x=w545) -> (x+1=w544:u32)
                  n81 = Greater Or Equal To 0?(x=w537) -> (x >= 0?=w547:bool)
                  n82 = Increment(x=w546) -> (x+1=w540:i32)
                  n83 = case shown="False" w547 {
                    tunnel: w544 -> [w554 _]
                    tunnel: w543 -> [w558 _]
                    tunnel: [w556 u8 6] -> w542
                    tunnel: [w555 u32 0] -> w541
                    tunnel: w540 -> [w553 w571]
                    tunnel: [w552 w571] -> w539
                    tunnel: w536 -> [w550 w570]
                    tunnel: [w551 w570] -> w535
                    tunnel: [w549 w569] -> w533
                    tunnel: w531 -> [w548 w569]
                    frame False {
                      n84 = Greater Or Equal?(x=w554, y=w558) -> (x >= y?=w557:bool)
                      n85 = case shown="True" w557 {
                        tunnel: [u8 5 u8 0] -> w556
                        tunnel: [w562 u32 0] -> w555
                        tunnel: w554 -> [w562 _]
                        tunnel: w553 -> [w561 _]
                        tunnel: [w561 0] -> w552
                        tunnel: [w560 0 ("High Correlation In")] -> w551
                        tunnel: w550 -> [w560 _]
                        tunnel: [w559 0 ("Old Average In")] -> w549
                        tunnel: w548 -> [w559 _]
                        frame False {
                        }
                        frame True {
                        }
                      }
                    }
                    frame True {
                    }
                  }
                }
                frame 6 {
                  n86 = Less?(x=w589, y=w576) -> (x < y?=w578:bool)
                  n87 = Greater Or Equal?(x=w589, y=w575) -> (x >= y?=w577:bool)
                  n88 = And(x=w578, y=w577) -> (x .and. y?=w588:bool)
                  n89 = case shown="True" w588 {
                    tunnel: [0 w606] -> w574
                    tunnel: w589 -> [_ w605]
                    tunnel: [w602 w605] -> w596
                    tunnel: w595 -> [w602 _]
                    tunnel: [u8 0 u8 7] -> w594
                    tunnel: [0 ("High Correlation In") w610] -> w593
                    tunnel: w592 -> [_ w610]
                    tunnel: [0 ("Old Average In") w609] -> w590
                    tunnel: w586 -> [_ w609]
                    frame False {
                    }
                    frame True {
                      n90 = Multiply(x=w605, y=fxp<+,6,1> 1.40625) -> (x*y=w604:fxp<+/-,38,33>)
                      n91 = To Long Integer(number=w604) -> (32bit integer=w603:i32)
                      n92 = Subtract(x=w603, y=19) -> (x-y=w606:i32)
                    }
                  }
                  n93 = Multiply(x=w574, y=w579) -> (x*y=w582:fxp<+/-,48,39>)
                  n94 = To Long Integer(number=w582) -> (32bit integer=w580:i32)
                }
                frame 7 {
                  n95 = Square(x=w620) -> (x^2=w616:i32)
                  n96 = Subtract(x=w635, y=w634) -> (x-y=w637:i32)
                  n97 = To Quad Integer(1:w616) -> (0:w629:i64)
                  n98 = Absolute Value(x=w637) -> (abs(x)=w615:i32)
                  n99 = To Quad Integer(1:w615) -> (0:w630:i64)
                  n100 = Greater Or Equal?(x=w640, y=w615) -> (x >= y?=w619:bool)
                  n101 = Less Or Equal?(x=w641, y=w615) -> (x <= y?=w618:bool)
                  n102 = Multiply(x=w630, y=w629) -> (x*y=w631:i64)
                  n103 = Greater Or Equal?(x=w620, y=w642) -> (x >= y?=w617:bool)
                  n104 = Less Or Equal?(x=w620, y=w643) -> (x <= y?=w614:bool)
                  n105 = Less Or Equal?(x=w631, y=w633) -> (x <= y?=w612:bool)
                  n106 = Greater Or Equal?(x=w631, y=w632) -> (x >= y?=w613:bool)
                  n107 = Compound Arithmetic op=AND(w619, w618, w617, w614, w612, w613) -> (w636:bool)
                  n108 = case shown="True" w636 {
                    tunnel: w646 -> [_ w656]
                    tunnel: [0 w654] -> w645
                    tunnel: [u8 0 u8 8] -> w644
                    tunnel: w639 -> [_ w655]
                    tunnel: [0 ("High Correlation In") w655] -> w638
                    tunnel: w628 -> [_ w652]
                    tunnel: [0 w651] -> w627
                    frame False {
                    }
                    frame True {
                      n109 = Decrement(x=w656) -> (x-1=w654:i32)
                      n110 = Decrement(x=w652) -> (x-1=w651:i32)
                    }
                  }
                }
                frame 8 {
                  n111 = Decrement(x=w675) -> (x-1=w676:i32)
                  n112 = Subtract(x=w663, y=w664) -> (x-y=w666:i32)
                  n113 = Less Or Equal To 0?(x=w676) -> (x <= 0?=w658:bool)
                  n114 = Absolute Value(x=w666) -> (abs(x)=w665:i32)
                  n115 = case shown="True" w658 {
                    tunnel: [u8 8 u8 9] -> w674
                    tunnel: [w680 w686] -> w673
                    tunnel: w659 -> [_ w684]
                    tunnel: w676 -> [w680 _]
                    tunnel: w670 -> [w678 _]
                    tunnel: [w678 w684] -> w669
                    tunnel: [w677 w683] -> w668
                    tunnel: w667 -> [w677 _]
                    tunnel: w665 -> [_ w683]
                    frame False {
                    }
                    frame True {
                      n116 = To Fixed-Point(number=w684) -> (fixed-point=w681:fxp<+/-,32,32>)  [unwired: 1 in]
                      n117 = Multiply(x=fxp<+,2,1> 1.5, y=w681) -> (x*y=w687:fxp<+/-,34,33>)
                      n118 = To Long Integer(number=w687) -> (32bit integer=w686:i32)
                    }
                  }
                  n119 = Decrement(x=w662) -> (x-1=w660:i32)
                  n120 = Less Or Equal To 0?(x=w660) -> (x <= 0?=w657:bool)
                }
                frame 9 {
                  n121 = Decrement(x=w705) -> (x-1=w702:i32)
                  n122 = Less Or Equal To 0?(x=w702) -> (x <= 0?=w691:bool)
                  n123 = case shown="True" w691 {
                    tunnel: [w708 0] -> w703
                    tunnel: [u8 9 u8 12] -> w704
                    tunnel: w702 -> [w708 _]
                    tunnel: w699 -> [w707 _]
                    tunnel: [w707 0 ("Noise Level")] -> w700
                    tunnel: [u16 0 u16 550] -> w692
                    frame False {
                    }
                    frame True {
                    }
                  }
                  n124 = Decrement(x=w693) -> (x-1=w688:i32)
                  n125 = Not(x=w691) -> (.not. x?=w690:bool)
                  n126 = Less Or Equal To 0?(x=w688) -> (x <= 0?=w689:bool)
                }
                frame 12 {
                  n127 = Decrement(x=w718) -> (x-1=w714:i32)
                  n128 = Less Or Equal To 0?(x=w714) -> (x <= 0?=w717:bool)
                  n129 = case shown="True" w717 {
                    tunnel: [FALSE w735] -> w719
                    tunnel: [u8 12 w740] -> w729
                    tunnel: w716 -> [w733 w741]
                    tunnel: [w733 w739] -> w728
                    tunnel: [w731 0] -> w715
                    tunnel: w714 -> [w731 _]
                    frame False {
                    }
                    frame True {
                      n130 = Decrement(x=w741) -> (x-1=w738:i32)
                      n131 = Less Or Equal To 0?(x=w738) -> (x <= 0?=w736:bool)
                      n132 = case shown="False" w736 {
                        tunnel: [u8 12 u8 0] -> w740
                        tunnel: [w742 u16 0] -> w739
                        tunnel: w738 -> [w742 _]
                        frame False {
                        }
                        frame True {
                        }
                      }
                      n133 = Not(x=w736) -> (.not. x?=w735:bool)
                    }
                  }
                }
              }
            }
            n134 = Or Array Elements(Boolean array=w189) -> (logical OR=w184:bool)
            n135 = Or Array Elements(Boolean array=w190) -> (logical OR=w188:bool)
            n136 = case shown="True" "One Shot" {
              tunnel: [w213 w219] -> w181
              tunnel: w184 -> [w213 w216]
              tunnel: [FALSE w221] -> w180
              tunnel: w182 -> [_ w215]
              frame False {
              }
              frame True {
                n137 = local read "Reset One Shot"() -> (w214:bool)
                n138 = local read "Armed"() -> (w222:bool)
                n139 = Or(x=w222, y=w214) -> (x .or. y?=w220:bool)
                n140 = Not(x=w215) -> (.not. x?=w217:bool)
                n141 = And(x=w220, y=w216) -> (x .and. y?=w219:bool)
                n142 = Or(x=w216, y=w217) -> (x .or. y?=w218:bool)
                n143 = And(x=w220, y=w218) -> (x .and. y?=w221:bool)
              }
            }
            "Delay" <- w181
            "Del Armed" <- w180
            n144 = case shown="True" "One Shot" {
              tunnel: [w224 w229] -> w185
              tunnel: w188 -> [w224 w226]
              tunnel: [FALSE w231] -> w187
              tunnel: w186 -> [_ w225]
              frame False {
              }
              frame True {
                n145 = local read "Armed"() -> (w233:bool)
                n146 = Or(x=w233, y="Reset One Shot") -> (x .or. y?=w230:bool)
                n147 = And(x=w230, y=w226) -> (x .and. y?=w229:bool)
                n148 = Not(x=w225) -> (.not. x?=w227:bool)
                n149 = Or(x=w226, y=w227) -> (x .or. y?=w228:bool)
                n150 = And(x=w230, y=w228) -> (x .and. y?=w231:bool)
              }
            }
            "Plates" <- w185
            "Armed" <- w187
            n151 = Array To Cluster(array=w210) -> (cluster=w121:T1)
            n152 = Array To Cluster(array=w208) -> (cluster=w120:T5)
            n153 = Array To Cluster(array=w197) -> (cluster=w119:T1)
            n154 = Array To Cluster(array=w196) -> (cluster=w118:T1)
            n155 = Array To Cluster(array=w195) -> (cluster=w117:T7)
            n156 = Array To Cluster(array=w194) -> (cluster=w116:T1)
            n157 = Array To Cluster(array=w193) -> (cluster=w115:T1)
            n158 = Array To Cluster(array=w192) -> (cluster=w114:T1)
            n159 = Array To Cluster(array=w191) -> (cluster=w113:T1)
            n160 = Array To Cluster(array=w205) -> (cluster=w112:T1)
            n161 = Array To Cluster(array=w206) -> (cluster=w111:T1)
          }
        }
        "New Average" <- w29
      }
      n162 = node-c288(refnum<k21> "IO Module\\Data Clock" ("Source Name")) -> (w8:T2)
      n163 = timed-loop {
        timing: w8 -> [_]
        timing-out: [_] -> w7
        stop <- _ stop-if-true
        n164 = xnode "FPGA I/O Node"() -> ("IO Module\\AI 1"=→"IO Module\\AI 1":i16)  [unwired: 1 in, 1 out]
        n165 = xnode "FPGA I/O Node"() -> ("IO Module\\AI 0"=→"IO Module\\AI 0":i16)  [unwired: 1 in, 1 out]
      }
      n166 = node-c288(w7) -> ()
      n167 = while {
        stop <- FALSE stop-if-true
        w28 = TRUE ("IO Module\\PFI Enable")
        n168 = local read "Plates"() -> (w26:bool)
        n169 = local read "Delay"() -> (w25:bool)
        n170 = xnode "FPGA I/O Node"("IO Module\\PFI 0 WE"=w28, "IO Module\\PFI 1 WE"=w28) -> ()  [unwired: 2 in, 2 out]
        n171 = xnode "FPGA I/O Node"("IO Module\\PFI 0 Wr Data"=w26, "IO Module\\PFI 1 Wr Data"=w25) -> ()  [unwired: 2 in, 2 out]
      }
      n172 = node-c288(w10) -> ()
    }
  }
